vi "Beam Detection-v6.vi"(0 "Image Src":T1, 3 "Pretreatment":bool, 4 "DetectionParameters":T5={"Contrast"=0, "Treshold"=60, "Peak Intensity"=0, "Peak Intensity%"=0, "Rx"=378, "Ry"=294, "R%"=294} {"Peak Intensity%" max=100 step=1}, 5 "error in":errorcluster, 7 "Display":T7) -> (13 "Ellipse":T3 {"Minor Axis"."Point 2"."Y" format="%.2f"; "Minor Axis"."Point 2"."X" format="%.2f"; "Minor Axis"."Point 1"."Y" format="%.2f"; "Minor Axis"."Point 1"."X" format="%.2f"; "Major Axis"."Point 2"."Y" format="%.2f"; "Major Axis"."Point 2"."X" format="%.2f"; "Major Axis"."Point 1"."Y" format="%.2f"; "Major Axis"."Point 1"."X" format="%.2f"; "Center"."Y" format="%.2f"; "Center"."X" format="%.2f"}, 14 "Image Out":T1, 15 "Beam is IN":bool, 16 "Ellipse edges":cluster{"X":sgl, "Y":sgl}[](array[cluster]), 17 "Best Rectangle":T2 {"Rotation" format="%.2f"; "Left" scale=0.0..1024.0; "Right" scale=0.0..1024.0}, 18 "ImgData":T6={"X Intensity"=[], "Y Intensity"=[], "Max Intensity"=0, "Centroid"={"X"=0, "Y"=0}, "Radius"={"Rx"=239, "Ry"=288}}, 19 "error out":errorcluster)   [LabVIEW 2013]
uses:
  <vilib>/vision/Image Controls.llb/IMAQ Image.ctl
  <vilib>/vision/Measure.llb/Edge Options.ctl
  <vilib>/vision/Measure.llb/Edge Polarity.ctl
  <vilib>/vision/NI_Vision_Development_Module.lvlib
panel:
  in  "override beam center with centroid":bool=TRUE
  out "Centroid":cluster{"X Centroid":sgl, "Y Centroid":sgl} {"Y Centroid" format="%.2f"; "X Centroid" format="%.2f"}
  out "Maximal Value":sgl
  out "Biggest Object":T4
  out "Image Buffer":T1(plugin-control)
  # "Contrast specifies the threshold for the contrast of the edge. Only edges with a contrast greater than this value are used in the detection process. Contrast is defined as the difference between the average pixel intensity before the edge and the average pixel intensity after the edge. \nFilter width specifies the number of pixels that the VI averages to find the contrast at either side of the edge.\nSteepness specifies the slope of the edge. This value represents the number of pixels that correspond to the transition area of the edge.\nSubsampling Ratio specifies the number of pixels that separate two consecutive search lines of the rake."
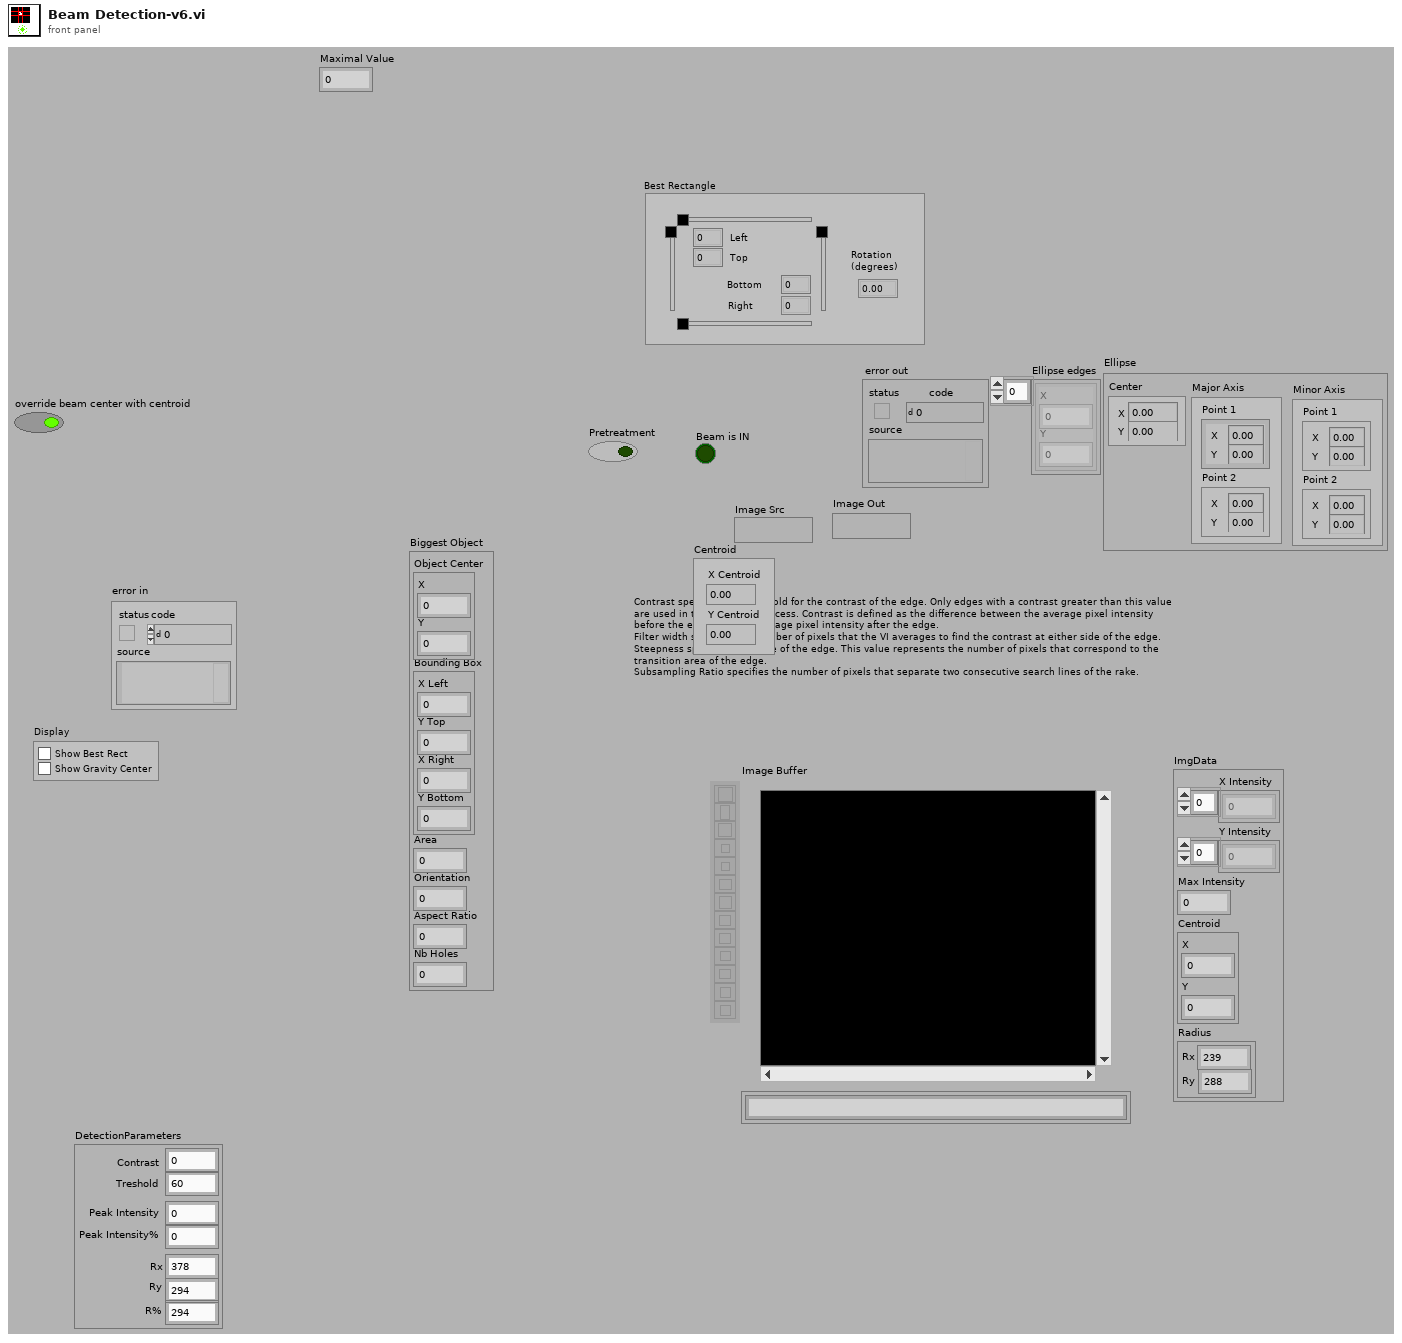
[diagram p1: front panel]
types:
  T1 = typedef "IMAQ Image.ctl" = refnum<image>
  T2 = typedef "IMAQ Rectangle" = cluster{"Left":i32, "Top":i32, "Right":i32, "Bottom":i32, "Rotation":dbl}
  T3 = cluster{"Center":cluster{"X":sgl, "Y":sgl}, "Major Axis":cluster{"Point 1":cluster{"X":sgl, "Y":sgl}, "Point 2":cluster{"X":sgl, "Y":sgl}}, "Minor Axis":cluster{"Point 1":cluster{"X":sgl, "Y":sgl}, "Point 2":cluster{"X":sgl, "Y":sgl}}}
  T4 = cluster{"Object Center":cluster{"X":sgl, "Y":sgl}, "Bounding Box":cluster{"X Left":i32, "Y Top":i32, "X Right":i32, "Y Bottom":i32}, "Area":sgl, "Orientation":sgl, "Aspect Ratio":sgl, "Nb Holes":i32}
  T5 = cluster{"Contrast":i32, "Treshold":u8, "Peak Intensity":i32, "Peak Intensity%":u8, "Rx":i32, "Ry":i32, "R%":i32}
  T6 = cluster{"X Intensity":u8[], "Y Intensity":u8[], "Max Intensity":u8, "Centroid":cluster{"X":i32, "Y":i32}, "Radius":cluster{"Rx":i32, "Ry":i32}}
  T7 = cluster{"Show Best Rect":bool, "Show Gravity Center":bool}
  T8 = enum32{"AutoM", "Close", "Dilate", "Erode", "Gradient", "Gradient in", "Gradient out", "HitMiss", "Open", "PClose", "POpen", "Thick", "Thin"}
  T9 = cluster{"Objects":u16, "Threshold":i32, "Reject Border":bool, "Fill Holes":bool, "Min Object Size":bool, "Min Size":i32, "Max Object Size":bool, "Max Size":i32, "Show Search Area":bool, "Show Center":bool, "Show Bounding Box":bool}
  T10 = enum16{"Get First Edge", "Get First + Last Edge", "Get All Edges", "Get Best Edge"}
  T11 = typedef "Edge Options.ctl" = cluster{"Edge Polarity":T12, "Kernel Size":u32, "Width":u32, "Minimum Edge Strength":sgl, "Interpolation Type":enum32{"Zero Order", "Bilinear", "Quadratic", "Cubic", "Bilinear Fixed"}, "Data Processing Method":enum32{"Average", "Median"}}
  T12 = typedef "Edge Polarity.ctl" = u32
  T13 = typedef "IMAQ Circle" = cluster{"Center X":i32, "Center Y":i32, "Inner Radius":i32, "Outer Radius":i32, "Start Angle":dbl, "End Angle":dbl}
  T14 = typedef "Image Type" = u32
  T15 = cluster{"Object Center":cluster{"X":sgl, "Y":sgl}, "Bounding Box":cluster{"X Left":i32, "Y Top":i32, "X Right":i32, "Y Bottom":i32}, "Area":sgl, "Orientation":sgl, "Aspect Ratio":sgl, "Nb Holes":i32}[]
  T16 = cluster{"histogram":u32[], "Minimal Value":sgl, "Maximal Value":sgl, "Starting Value":sgl, "Interval Width":sgl, "Mean Value":sgl, "Standard  Variation":sgl, "Area (pixels)":i32}
  T17 = cluster{"X Left":i32, "Y Top":i32, "X Right":i32, "Y Bottom":i32, "Orientation":sgl}
  T18 = typedef "ROI Descriptor" = cluster{"Global Rectangle":i32[], "Contours":cluster{"ID":enum32{"External", "Internal"}, "Type":u32, "Coordinates":i32[]}[]}
  T19 = typedef "Edge New.ctl" = cluster{"Location (Pixel)":cluster{"X":sgl, "Y":sgl}, "Location (Real-World)":cluster{"X":sgl, "Y":sgl}, "Distance (Pixel)":dbl, "Distance (Real-World)":dbl, "Strength":dbl, "Noise":dbl, "Rising?":bool}
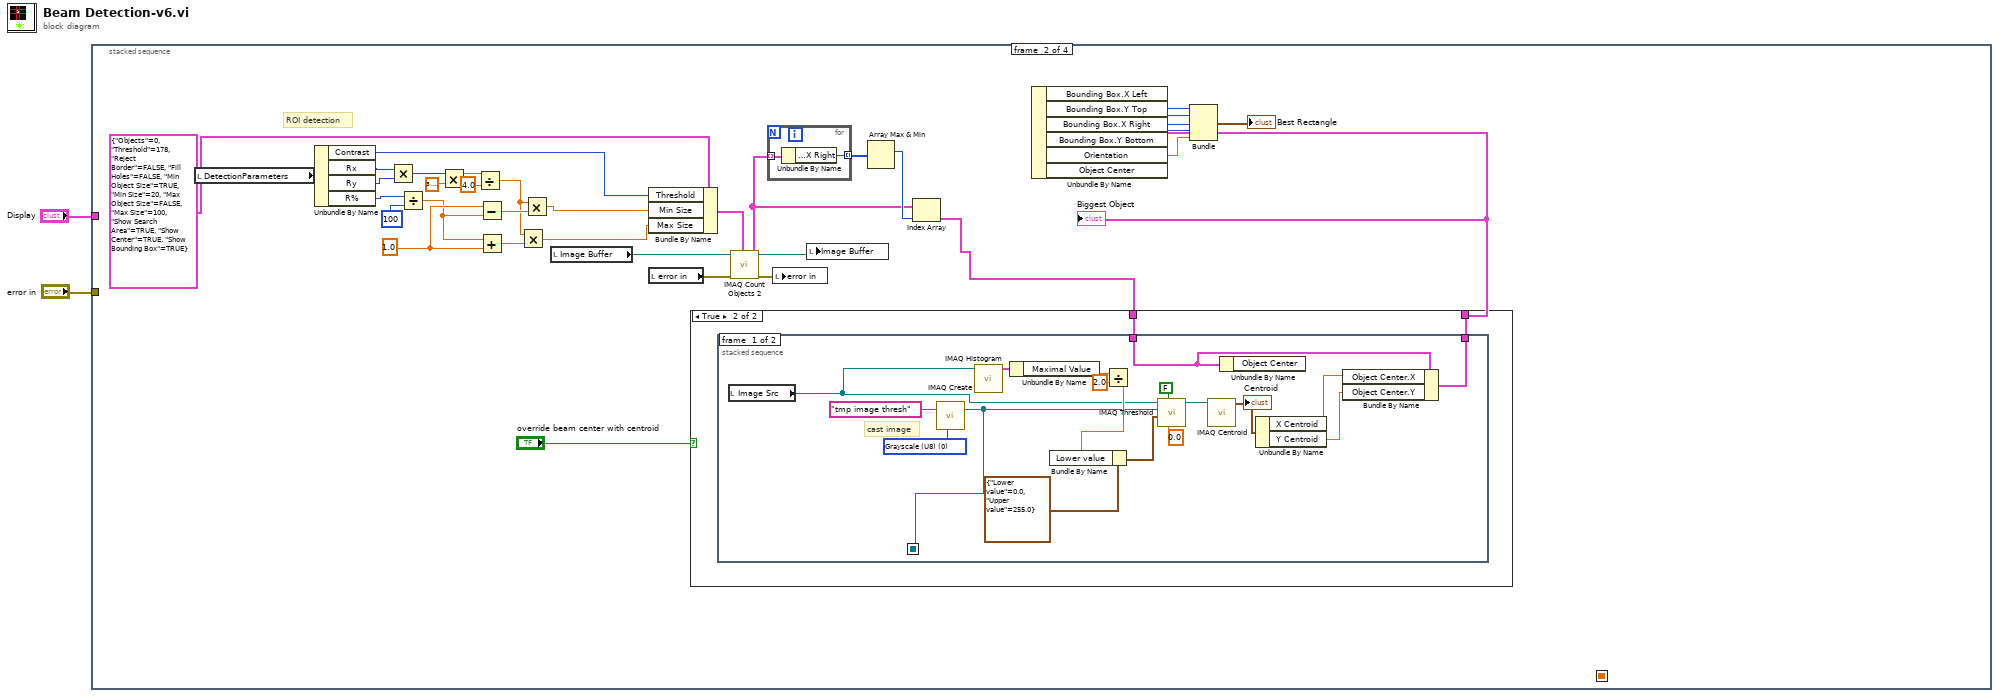
[diagram p0: block diagram]
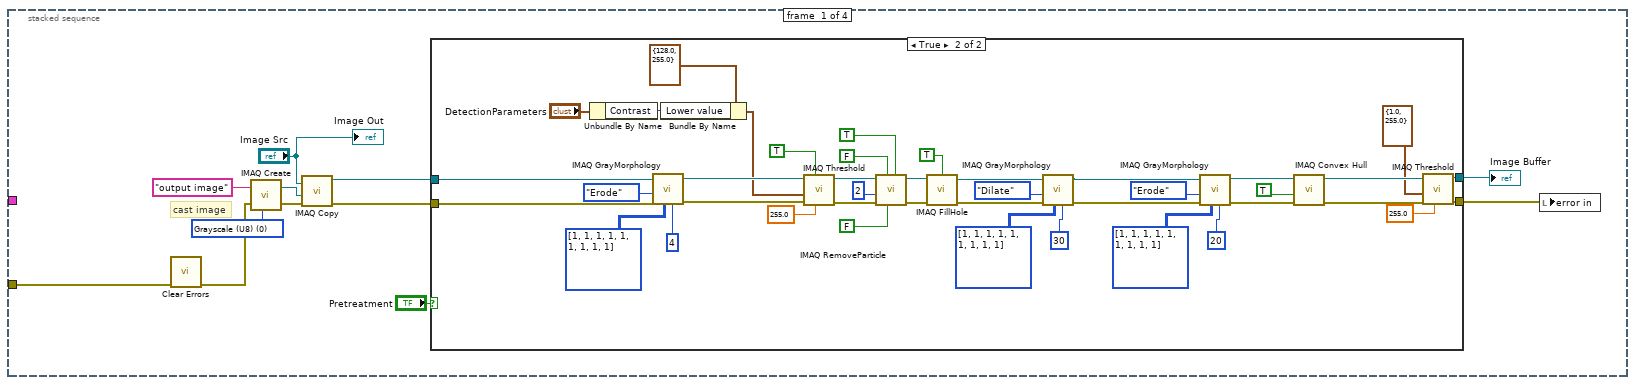
[diagram p2: hidden frame]
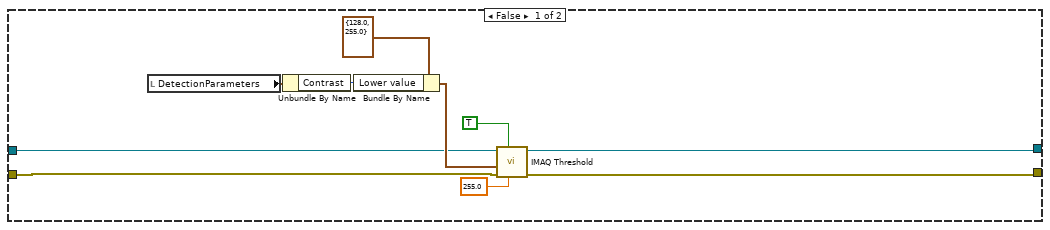
[diagram p3: hidden frame]
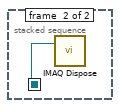
[diagram p5: hidden frame]
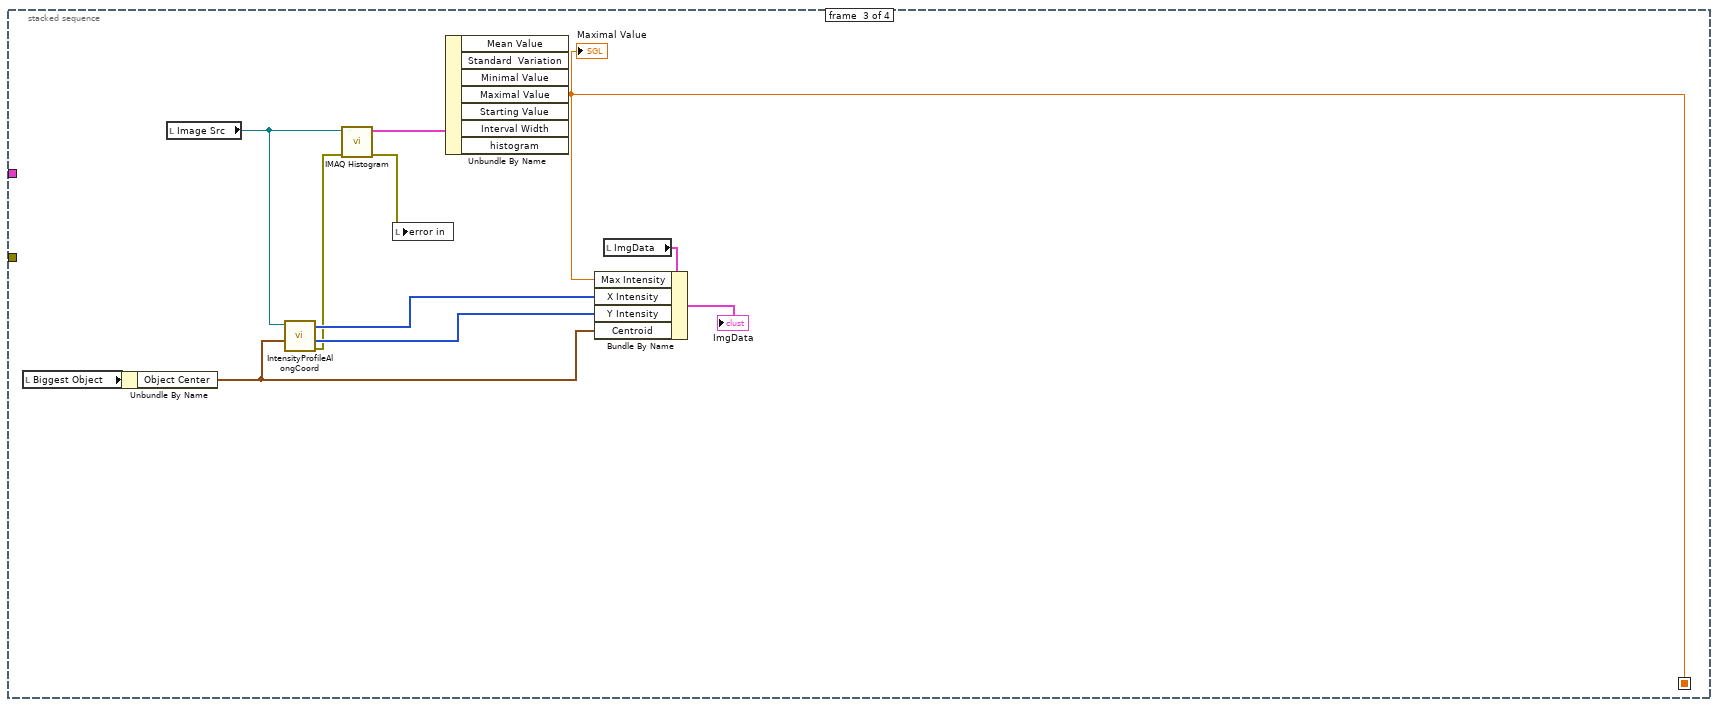
[diagram p6: hidden frame]
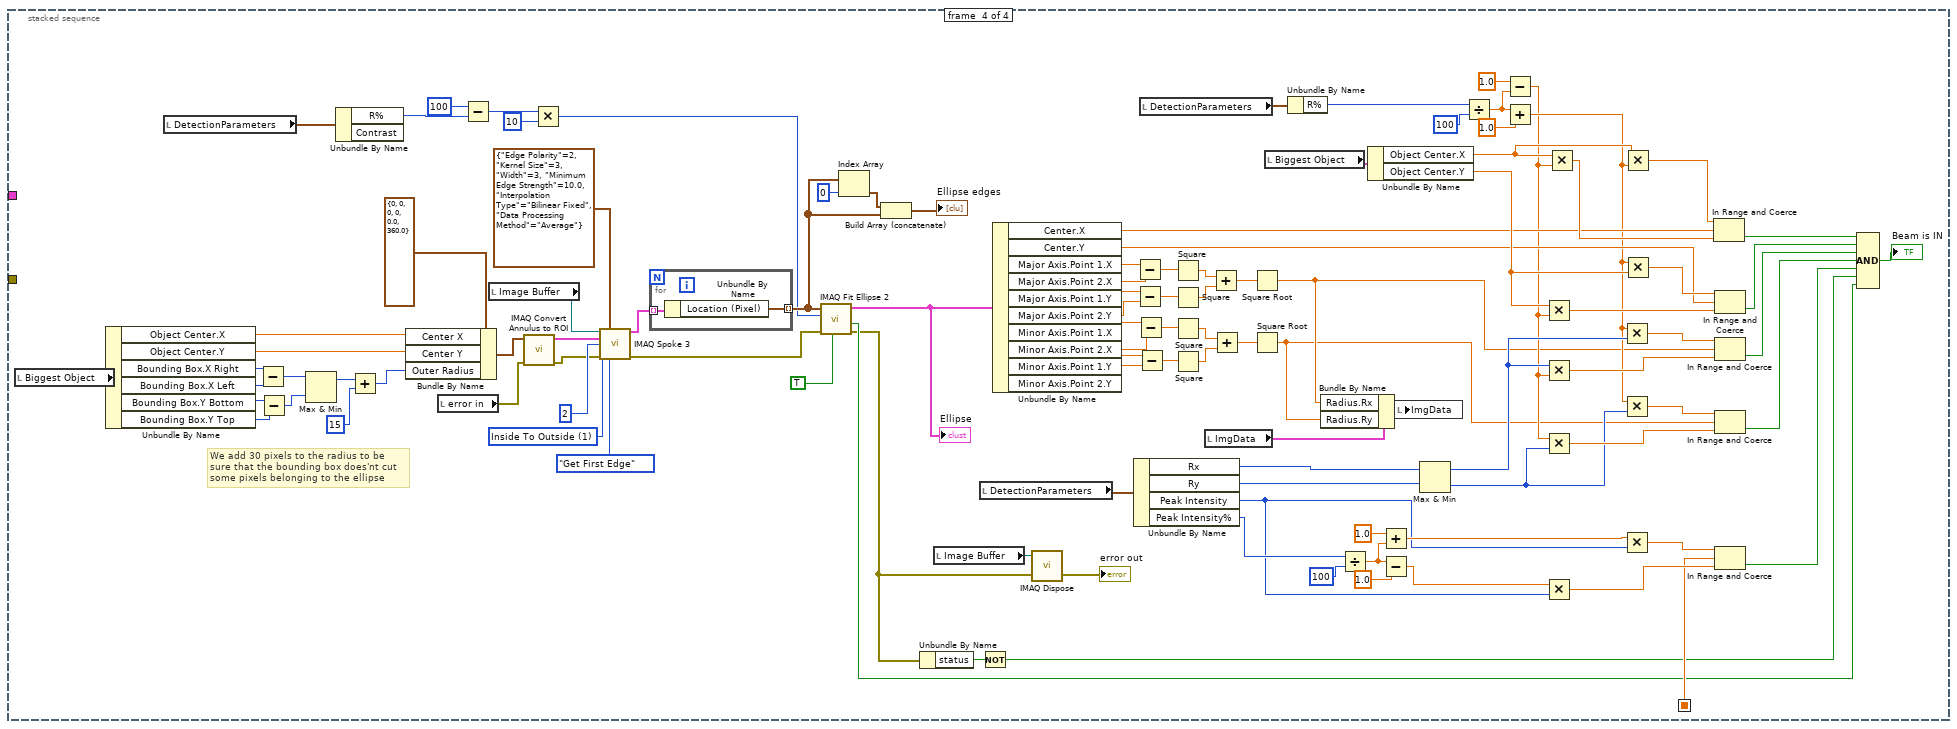
[diagram p7: hidden frame]
diagram:
  n1 = stacked-sequence {
    seq-local: [_ _ w128 _] -> [_ _ _ w151]
    tunnel: "Display" -> [_ _ _ _]
    tunnel: "error in" -> [w8 _ _ _]
    frame #0 {
      w11 = T14 0 items=["Grayscale (U8)", "Grayscale (I16)", "Grayscale (SGL)", "Complex (CSG)", "RGB (U32)", "HSL (U32)", "RGB (U64)", "Grayscale (U16)"] ("Image Type")
      # "cast image"
      n2 = call <vilib>:"Clear Errors.vi"("error in (no error)"=w8) -> ("error out"=w7:errorcluster)  [unwired: 6 in]
      n3 = call "IMAQ Create"("Image Name"="output image", "Image Type"=w11, "error in (no error)"=w7) -> ("New Image"=w12:T1, "error out"=w13:errorcluster)  [unwired: 2 in]
      n4 = call "IMAQ Copy"("error in (no error)"=w13, "Image Dst"=w12, "Image Src"="Image Src") -> ("error out"=w5:errorcluster, "Image Dst Out"=w6:T1)  [unwired: 3 in]
      n5 = case shown="True" "Pretreatment" {
        tunnel: [w16 w58] -> w10
        tunnel: [w15 w57] -> w9
        tunnel: w6 -> [w18 w46]
        tunnel: w5 -> [w17 w44]
        frame False {
          n6 = local read "DetectionParameters"() -> (w24:T5)
          n7 = Unbundle By Name(w24) -> ("Contrast"=w20:i32)
          n8 = Bundle By Name(cluster=cluster{"Lower value":sgl, "Upper value":sgl} {"Lower value"=128.0, "Upper value"=255.0} ("Range"), "Lower value"=w20) -> (w19:cluster{"Lower value":sgl, "Upper value":sgl})
          n9 = call "IMAQ Threshold"("Replace Value"=sgl 255.0, "Keep/Replace Value (Replace)"=TRUE, "error in (no error)"=w17, "Range"=w19, "Image Src"=w18) -> ("error out"=w15:errorcluster, "Image Dst Out"=w16:T1)  [unwired: 5 in]
        }
        frame True {
          n10 = Unbundle By Name("DetectionParameters") -> ("Contrast"=w26:i32)
          n11 = call "IMAQ GrayMorphology"("Number of iterations (1)"=4, "Structuring Element"=i32[][] [[1, 1, 1], [1, 1, 1], [1, 1, 1]], "error in (no error)"=w44, "Operation"=T8."Erode", "Image Src"=w46) -> ("error out"=w43:errorcluster, "Image Dst Out"=w45:T1)  [unwired: 2 in, 3 out]
          n12 = Bundle By Name(cluster=cluster{"Lower value":sgl, "Upper value":sgl} {"Lower value"=128.0, "Upper value"=255.0} ("Range"), "Lower value"=w26) -> (w25:cluster{"Lower value":sgl, "Upper value":sgl})
          n13 = call "IMAQ Threshold"("Replace Value"=sgl 255.0, "Keep/Replace Value (Replace)"=TRUE, "error in (no error)"=w43, "Range"=w25, "Image Src"=w45) -> ("error out"=w65:errorcluster, "Image Dst Out"=w60:T1)  [unwired: 5 in]
          n14 = call "IMAQ RemoveParticle"("Connectivity 4/8 (8)"=TRUE, "Low Pass/High Pass (Low)"=FALSE, "Square/Hexa (Square)"=FALSE, "error in (no error)"=w65, "Number of Erosion"=2, "Image Src"=w60) -> ("error out"=w50:errorcluster, "Image Dst Out"=w51:T1)  [unwired: 1 in, 3 out]
          n15 = call "IMAQ FillHole"("error in (no error)"=w50, "Image Src"=w51, "Connectivity 4/8 (8)"=TRUE) -> ("error out"=w38:errorcluster, "Image Dst Out"=w39:T1)  [unwired: 3 in]
          n16 = call "IMAQ GrayMorphology"("Number of iterations (1)"=30, "Structuring Element"=i32[][] [[1, 1, 1], [1, 1, 1], [1, 1, 1]], "error in (no error)"=w38, "Operation"=T8."Dilate", "Image Src"=w39) -> ("error out"=w33:errorcluster, "Image Dst Out"=w34:T1)  [unwired: 2 in, 3 out]
          n17 = call "IMAQ GrayMorphology"("Number of iterations (1)"=20, "Structuring Element"=i32[][] [[1, 1, 1], [1, 1, 1], [1, 1, 1]], "error in (no error)"=w33, "Operation"=T8."Erode", "Image Src"=w34) -> ("error out"=w32:errorcluster, "Image Dst Out"=w31:T1)  [unwired: 2 in, 3 out]
          n18 = call "IMAQ Convex Hull"("error in (no error)"=w32, "Connectivity 4/8 (8)"=TRUE, "Image Src"=w31) -> ("error out"=w55:errorcluster, "Image Dst Out"=w56:T1)  [unwired: 1 in, 6 out]
          n19 = call "IMAQ Threshold"("Replace Value"=sgl 255.0, "error in (no error)"=w55, "Range"=cluster{"Lower value":sgl, "Upper value":sgl} {"Lower value"=1.0, "Upper value"=255.0}, "Image Src"=w56) -> ("error out"=w57:errorcluster, "Image Dst Out"=w58:T1)  [unwired: 6 in]
        }
      }
      "Image Buffer" <- w10
      n20 = local write "error in"(w9) -> ()
      "Image Out" <- "Image Src"
    }
    frame #1 {
      w91 = 1.0 ("y")
      # "ROI detection"
      n21 = local read "DetectionParameters"() -> (w99:T5)
      n22 = Unbundle By Name(w99) -> ("Contrast"=w72:i32, "Rx"=w88:i32, "Ry"=w98:i32, "R%"=w97:i32)
      n23 = Multiply(x=w88, y=w98) -> (x*y=w85:i32)
      n24 = Divide(x=w97, y=100) -> (x/y=w90:dbl)
      n25 = Multiply(x=w85, y=3.141592653589793) -> (x*y=w74:dbl)
      n26 = Divide(x=w74, y=4.0) -> (x/y=w76:dbl)
      n27 = Subtract(x=w91, y=w90) -> (x-y=w89:dbl)
      n28 = Add(x=w90, y=w91) -> (x+y=w92:dbl)
      n29 = Multiply(x=w76, y=w92) -> (x*y=w77:dbl)
      n30 = Multiply(x=w76, y=w89) -> (x*y=w78:dbl)
      n31 = local read "Image Buffer"() -> (w69:T1)
      n32 = Bundle By Name(cluster=T9 {"Objects"=0, "Threshold"=178, "Reject Border"=FALSE, "Fill Holes"=FALSE, "Min Object Size"=TRUE, "Min Size"=20, "Max Object Size"=FALSE, "Max Size"=100, "Show Search Area"=TRUE, "Show Center"=TRUE, "Show Bounding Box"=TRUE} ("Settings"), "Threshold"=w72, "Min Size"=w78, "Max Size"=w77) -> (w87:T9)
      n33 = local read "error in"() -> (w95:errorcluster)
      n34 = call "IMAQ Count Objects 2"("Settings"=w87, "error in (no error)"=w95, "Image"=w69) -> ("error out"=w70:errorcluster, "Image Out"=w71:T1, "Objects"=w93:T15)  [unwired: 4 in, 2 out]
      n35 = for {
        tunnel: w93 -> [w124] mode=indexing
        tunnel: [w123] -> w86 mode=indexing
        n36 = Unbundle By Name(w124) -> ("Bounding Box.X Right"=w123:i32)
      }
      n37 = local write "error in"(w70) -> ()
      n38 = local write "Image Buffer"(w71) -> ()
      n39 = Array Max & Min(array=w86) -> (max index (indices)=w94:i32)  [unwired: 3 out]
      n40 = Index Array(array=w93, index=w94) -> (element=w68:T4)
      n41 = case shown="True" "override beam center with centroid" {
        tunnel: w68 -> [w101 w103]
        tunnel: [w101 w102] -> w67
        frame False {
        }
        frame True {
          n42 = stacked-sequence {
            seq-local: [w110 _] -> [_ w122]
            tunnel: w103 -> [w108 _]
            tunnel: [w104 _] -> w102
            frame #0 {
              w120 = T14 0 items=["Grayscale (U8)", "Grayscale (I16)", "Grayscale (SGL)", "Complex (CSG)", "RGB (U32)", "HSL (U32)", "RGB (U64)", "Grayscale (U16)"] ("Image Type")
              # "cast image"
              n43 = local read "Image Src"() -> (w111:T1)
              n44 = call "IMAQ Create"("Image Name"="tmp image thresh", "Image Type"=w120) -> ("New Image"=w110:T1)  [unwired: 3 in, 1 out]
              n45 = call "IMAQ Histogram"("Image"=w111) -> ("Histogram Report"=w118:T16)  [unwired: 4 in, 6 out]
              n46 = Unbundle By Name(w118) -> ("Maximal Value"=w116:sgl)
              n47 = Divide(x=w116, y=sgl 2.0) -> (x/y=w114:sgl)
              n48 = Bundle By Name(cluster=cluster{"Lower value":sgl, "Upper value":sgl} {"Lower value"=0.0, "Upper value"=255.0} ("Range"), "Lower value"=w114) -> (w113:cluster{"Lower value":sgl, "Upper value":sgl})
              n49 = call "IMAQ Threshold"("Replace Value"=sgl 0.0, "Keep/Replace Value (Replace)"=FALSE, "Range"=w113, "Image Dst"=w110, "Image Src"=w111) -> ("Image Dst Out"=w112:T1)  [unwired: 5 in, 1 out]
              n50 = call "IMAQ Centroid"("Image"=w112) -> ("Centroid"=w107:cluster{"X Centroid":sgl, "Y Centroid":sgl})  [unwired: 3 in, 1 out]
              "Centroid" <- w107
              n51 = Unbundle By Name(w108) -> ()  [unwired: 1 out]
              n52 = Unbundle By Name(w107) -> ("X Centroid"=w106:sgl, "Y Centroid"=w105:sgl)
              n53 = Bundle By Name(cluster=w108, "Object Center.X"=w106, "Object Center.Y"=w105) -> (w104:T4)
            }
            frame #1 {
              n54 = call "IMAQ Dispose"("Image"=w122) -> ()  [unwired: 5 in, 1 out]
            }
          }
        }
      }
      "Biggest Object" <- w67
      n55 = Unbundle By Name(w67) -> ("Bounding Box.X Left"=w84:i32, "Bounding Box.Y Top"=w83:i32, "Bounding Box.X Right"=w82:i32, "Bounding Box.Y Bottom"=w81:i32, "Orientation"=w80:sgl)  [unwired: 1 out]
      n56 = Bundle("X Left"=w84, "Y Top"=w83, "X Right"=w82, "Y Bottom"=w81, "Orientation"=w80) -> (→"Best Rectangle":T17)  [unwired: 1 in]
    }
    frame #2 {
      n57 = local read "Biggest Object"() -> (w133:T4)
      n58 = Unbundle By Name(w133) -> ("Object Center"=w132:cluster{"X":sgl, "Y":sgl})
      n59 = local read "Image Src"() -> (w125:T1)
      n60 = call "IntensityProfileAlongCoord.vi"("Coord"=w132, "Image Src"=w125) -> ("error out"=w126:errorcluster, "Y Intensity (U8)"=w130:u8[], "X Intensity (U8)"=w131:u8[])  [unwired: 4 in, 3 out]
      n61 = call "IMAQ Histogram"("error in (no error)"=w126, "Image"=w125) -> ("error out"=w127:errorcluster, "Histogram Report"=w129:T16)  [unwired: 3 in, 5 out]
      n62 = local write "error in"(w127) -> ()
      n63 = Unbundle By Name(w129) -> ("Maximal Value"=w128:sgl)  [unwired: 6 out]
      "Maximal Value" <- w128
      n64 = local read "ImgData"() -> (w135:T6)
      n65 = Bundle By Name(cluster=w135, "Max Intensity"=w128, "X Intensity"=w131, "Y Intensity"=w130, "Centroid"=w132) -> (→"ImgData":T6)
    }
    frame #3 {
      w199 = u16 1 items=["Outside To Inside", "Inside To Outside"] ("Scan Direction")
      # "We add 30 pixels to the radius to be sure that the bounding box does'nt cut some pixels belonging to the ellipse"
      n66 = local read "Biggest Object"() -> (w218:T4)
      n67 = Unbundle By Name(w218) -> ("Object Center.X"=w215:sgl, "Object Center.Y"=w214:sgl, "Bounding Box.X Right"=w213:i32, "Bounding Box.X Left"=w212:i32, "Bounding Box.Y Bottom"=w211:i32, "Bounding Box.Y Top"=w210:i32)
      n68 = local read "DetectionParameters"() -> (w242:T5)
      n69 = Subtract(x=w213, y=w212) -> (x-y=w209:i32)
      n70 = Subtract(x=w211, y=w210) -> (x-y=w208:i32)
      n71 = Max & Min(x=w209, y=w208) -> (max(x,y)=w206:i32)  [unwired: 1 out]
      n72 = Unbundle By Name(w242) -> ("R%"=w241:i32)  [unwired: 1 out]
      n73 = Add(x=w206, y=15) -> (x+y=w207:i32)
      n74 = Bundle By Name(cluster=T13 {"Center X"=0, "Center Y"=0, "Inner Radius"=0, "Outer Radius"=0, "Start Angle"=0.0, "End Angle"=360.0} ("Annulus"), "Center X"=w215, "Center Y"=w214, "Outer Radius"=w207) -> (w217:T13)
      n75 = local read "error in"() -> (w198:errorcluster)
      n76 = Subtract(x=100, y=w241) -> (x-y=w239:i32)
      n77 = local read "Image Buffer"() -> (w204:T1)
      n78 = call "IMAQ Convert Annulus to ROI"("error in (no error)"=w198, "Annulus"=w217) -> ("error out"=w197:errorcluster, "ROI Descriptor"=w203:T18)  [unwired: 7 in]
      n79 = Multiply(x=w239, y=10) -> (x*y=w147:i32)
      n80 = call "IMAQ Spoke 3"("Image"=w204, "Edge Options"=T11 {"Edge Polarity"=2, "Kernel Size"=3, "Width"=3, "Minimum Edge Strength"=10.0, "Interpolation Type"=enum."Bilinear Fixed", "Data Processing Method"=enum."Average"}, "ROI Descriptor"=w203, "Step Size"=u32 2, "Scan Direction"=w199, "error in (no error)"=w197, "Process"=T10."Get First Edge") -> ("First Edges"=w196:T19[], "error out"=w195:errorcluster)  [unwired: 5 in, 2 out]
      n81 = for {
        tunnel: w196 -> [w244] mode=indexing
        tunnel: [w243] -> w192 mode=indexing
        n82 = Unbundle By Name(w244) -> ("Location (Pixel)"=w243:cluster{"X":sgl, "Y":sgl})
      }
      n83 = call "IMAQ Fit Ellipse 2"("Reject Outliers (FALSE)"=TRUE, "error in (no error)"=w195, "Minimum Score"=w147, "Radial Points"=w192) -> ("error out"=w140:errorcluster, "Valid Fit"=w150:bool, "Ellipse"=w143:T3)  [unwired: 2 in, 3 out]
      "Ellipse" <- w143
      n84 = Index Array(array=w192, index=0) -> (element=w146:cluster{"X":sgl, "Y":sgl})
      n85 = Build Array (concatenate)(w146, w192) -> (→"Ellipse edges":cluster{"X":sgl, "Y":sgl}[])
      n86 = Unbundle By Name(w140) -> ("status"=w194:bool)
      n87 = local read "Image Buffer"() -> (w142:T1)
      n88 = local read "DetectionParameters"() -> (w173:T5)
      n89 = Not(x=w194) -> (.not. x?=w149:bool)
      n90 = Unbundle By Name(w143) -> ("Center.X"=w170:sgl, "Center.Y"=w169:sgl, "Major Axis.Point 1.X"=w190:sgl, "Major Axis.Point 2.X"=w191:sgl, "Major Axis.Point 1.Y"=w189:sgl, "Major Axis.Point 2.Y"=w188:sgl, "Minor Axis.Point 1.X"=w187:sgl, "Minor Axis.Point 2.X"=w186:sgl, "Minor Axis.Point 1.Y"=w185:sgl, "Minor Axis.Point 2.Y"=w184:sgl)
      n91 = call "IMAQ Dispose"("Image"=w142, "error in (no error)"=w140) -> ("error out"=→"error out":errorcluster)  [unwired: 4 in]
      n92 = Unbundle By Name(w173) -> ("Rx"=w172:i32, "Ry"=w171:i32, "Peak Intensity"=w152:i32, "Peak Intensity%"=w155:u8)
      n93 = Subtract(x=w190, y=w191) -> (x-y=w183:sgl)
      n94 = Subtract(x=w189, y=w188) -> (x-y=w182:sgl)
      n95 = Subtract(x=w187, y=w186) -> (x-y=w181:sgl)
      n96 = Subtract(x=w185, y=w184) -> (x-y=w180:sgl)
      n97 = local read "DetectionParameters"() -> (w237:T5)
      n98 = Square(x=w183) -> (x^2=w179:sgl)
      n99 = Square(x=w182) -> (x^2=w177:sgl)
      n100 = Square(x=w181) -> (x^2=w178:sgl)
      n101 = Square(x=w180) -> (x^2=w176:sgl)
      n102 = local read "ImgData"() -> (w139:T6)
      n103 = Add(x=w179, y=w177) -> (x+y=w175:sgl)
      n104 = Add(x=w178, y=w176) -> (x+y=w174:sgl)
      n105 = Square Root(x=w175) -> (sqrt(x)=w137:sgl)
      n106 = Square Root(x=w174) -> (sqrt(x)=w136:sgl)
      n107 = local read "Biggest Object"() -> (w236:T4)
      n108 = Unbundle By Name(w237) -> ("R%"=w235:i32)
      n109 = Bundle By Name(cluster=w139, "Radius.Rx"=w137, "Radius.Ry"=w136) -> (w138:T6)
      n110 = Divide(x=w155, y=100) -> (x/y=w158:dbl)
      n111 = Unbundle By Name(w236) -> ("Object Center.X"=w226:sgl, "Object Center.Y"=w223:sgl)
      n112 = Add(x=1.0 ("y"), y=w158) -> (x+y=w154:dbl)
      n113 = Subtract(x=w158, y=1.0) -> (x-y=w153:dbl)
      n114 = local write "ImgData"(w138) -> ()
      n115 = Max & Min(x=w172, y=w171) -> (max(x,y)=w166:i32, min(x,y)=w165:i32)
      n116 = Divide(x=w235, y=100) -> (x/y=w232:dbl)
      n117 = Subtract(x=1.0 ("y"), y=w232) -> (x-y=w160:dbl)
      n118 = Add(x=w232, y=1.0) -> (x+y=w161:dbl)
      n119 = Multiply(x=w223, y=w160) -> (x*y=w224:dbl)
      n120 = Multiply(x=w166, y=w160) -> (x*y=w220:dbl)
      n121 = Multiply(x=w160, y=w165) -> (x*y=w168:dbl)
      n122 = Multiply(x=w153, y=w152) -> (x*y=w162:dbl)
      n123 = Multiply(x=w226, y=w160) -> (x*y=w227:dbl)
      n124 = Multiply(x=w161, y=w166) -> (x*y=w221:dbl)
      n125 = Multiply(x=w161, y=w165) -> (x*y=w167:dbl)
      n126 = Multiply(x=w154, y=w152) -> (x*y=w163:dbl)
      n127 = Multiply(x=w226, y=w161) -> (x*y=w225:dbl)
      n128 = Multiply(x=w161, y=w223) -> (x*y=w222:dbl)
      n129 = In Range and Coerce(upper limit=w225, x=w170, lower limit=w227) -> (In Range?=w230:bool)  [unwired: 1 out]
      n130 = In Range and Coerce(upper limit=w222, x=w169, lower limit=w224) -> (In Range?=w229:bool)  [unwired: 1 out]
      n131 = In Range and Coerce(upper limit=w221, x=w137, lower limit=w220) -> (In Range?=w228:bool)  [unwired: 1 out]
      n132 = In Range and Coerce(upper limit=w167, x=w136, lower limit=w168) -> (In Range?=w164:bool)  [unwired: 1 out]
      n133 = In Range and Coerce(upper limit=w163, x=w151, lower limit=w162) -> (In Range?=w148:bool)  [unwired: 1 out]
      n134 = Compound Arithmetic op=AND(w230, w229, w228, w164, w148, w149, w150) -> (→"Beam is IN":bool)
    }
  }
